vi "Even Bit Extractor (SubVI).vi"(10 "loop Index":i8, 11 "Input PN sequence":i8[](array[numeric])) -> (3 "Even Bits":i8)   [LabVIEW 2026]
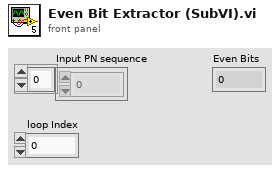
[diagram p1: front panel]
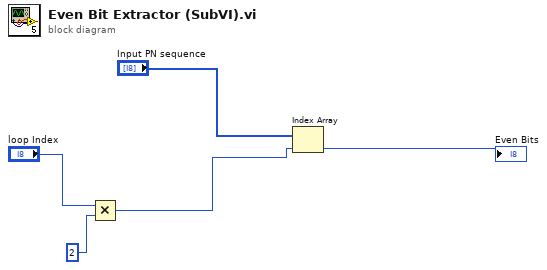
[diagram p0: block diagram]
diagram:
  n1 = Multiply(x="loop Index", y=i8 2) -> (x*y=w4:i8)
  n2 = Index Array(array="Input PN sequence", index=w4) -> (element=→"Even Bits":i8)
